vi "latitude.vi"() -> ()   [LabVIEW 2015]
panel:
  in  "latitude":dbl
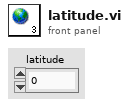
[diagram p1: front panel]
diagram:
